vi "Read XPS Init file.vi"(8 "error in":errorcluster, 11 "refnum in":T2 caption="refnum") -> (0 "error out":errorcluster, 2 "MHL Configuration":T1, 3 "refnum out":T2 caption="refnum en sortie")   [LabVIEW 2013, in "Data Configuration File.lvlib"]
doc: "Ce VI Récupère les donnée de configuration de la platine XY. Il permet la définition des limite de déplacement et de vitesse à utiliser avec la platine."
uses:
  Data Configuration File.lvlib
  <vilib>/Utility/config.llb/Config Data RefNum.ctl
  MHL configuration.ctl
  <vilib>/Utility/config.llb/Read Key (Double).vi
  <vilib>/Utility/config.llb/NI_LVConfig.lvlib
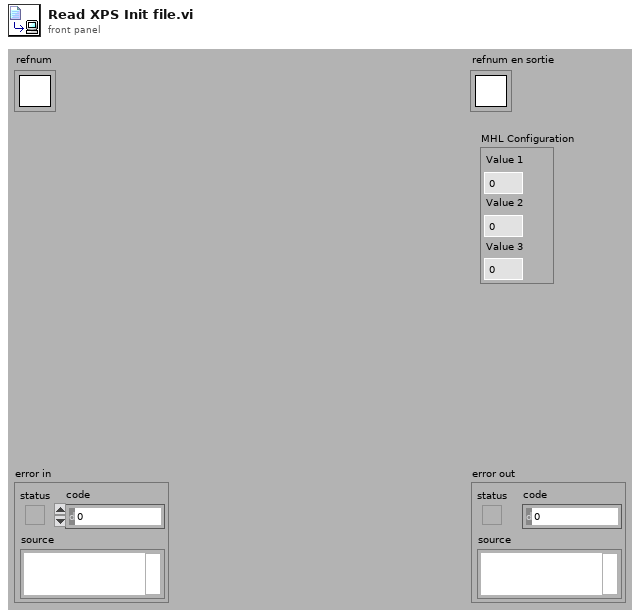
[diagram p1: front panel]
types:
  T1 = typedef "Data Configuration File.lvlib/MHL configuration.ctl" = cluster{"Value 1":dbl, "Value 2":dbl, "Value 3":dbl}
  T2 = typedef "NI_LVConfig.lvlib/Config Data RefNum.ctl" = refnum<k1>
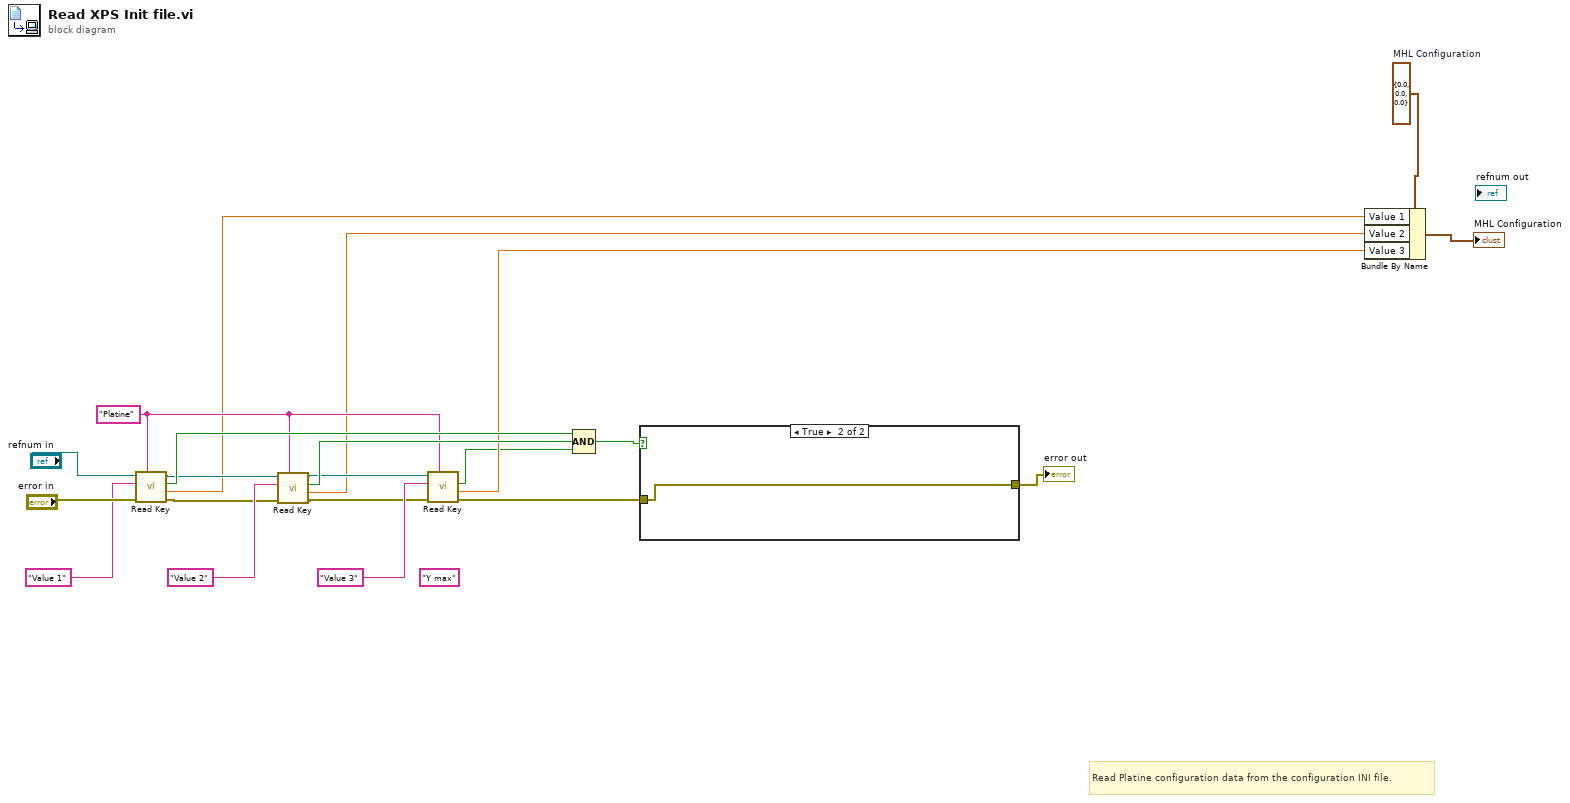
[diagram p0: block diagram]
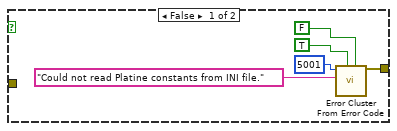
[diagram p2: hidden frame]
diagram:
  w4 = T1 {"Value 1"=0.0, "Value 2"=0.0, "Value 3"=0.0}  # MHL Configuration
  (unwired) "Y max"
  w8 = "Platine" ("section")
  # "Read Platine configuration data from the configuration INI file."
  n1 = call-poly <vilib>:"Read Key.vi"("section"=w8, "error in (no error)"="error in", "key"="Value 1", "refnum"="refnum in") -> ("error out"=w14:errorcluster, "value"=w2:dbl, "found?"=w16:bool, "refnum out"=w13:T2)  [unwired: 4 in]
  n2 = call-poly <vilib>:"Read Key.vi"("section"=w8, "error in (no error)"=w14, "key"="Value 2", "refnum"=w13) -> ("error out"=w10:errorcluster, "value"=w7:dbl, "found?"=w12:bool, "refnum out"=w9:T2)  [unwired: 4 in]
  n3 = call-poly <vilib>:"Read Key.vi"("section"=w8, "error in (no error)"=w10, "key"="Value 3", "refnum"=w9) -> ("error out"=w3:errorcluster, "value"=w6:dbl, "found?"=w5:bool)  [unwired: 4 in, 1 out]
  n4 = Compound Arithmetic op=AND(w16, w12, w5) -> (w19:bool)
  n5 = case shown="True" w19 {
    tunnel: [w26 w27] -> w21
    tunnel: w3 -> [_ w27]
    frame False {
      n6 = call <vilib>:"Error Cluster From Error Code.vi"("is warning? (False)"=FALSE, "show call chain? (False)"=TRUE, "error message (\"\")"="Could not read Platine constants from INI file." ("error message (\"\")"), "error code (0)"=5001) -> ("error out"=w26:errorcluster)  [unwired: 5 in]
    }
    frame True {
    }
  }
  "error out" <- w21
  n7 = Bundle By Name(cluster=w4, "Value 1"=w2, "Value 2"=w7, "Value 3"=w6) -> (→"MHL Configuration":T1)
